vi "SendRawCommand.vi"(8 "Error In":errorcluster, 10 "Command":string, 11 "VISA resource name":refnum<visa-resource-name>) -> (0 "Error Out":errorcluster, 3 "VISA resource name out":refnum<visa-resource-name>)   [LabVIEW 2019, in "Mark 10 TSTM-DC.lvlib"]
uses:
  Mark 10 TSTM-DC.lvlib
  Mark 10 Event Monitor/Mark 10 Event Monitor.lvlib
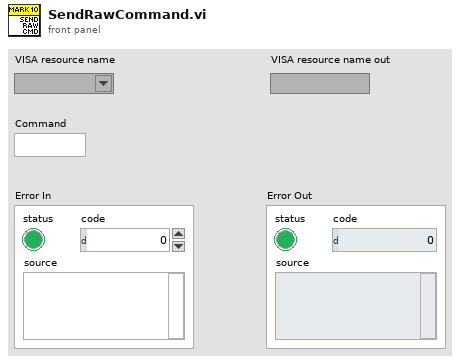
[diagram p1: front panel]
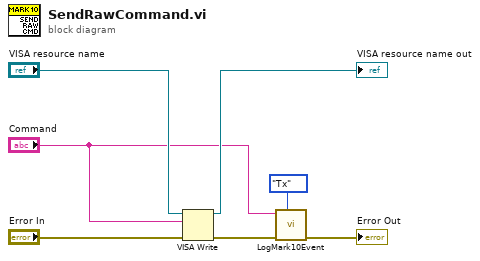
[diagram p0: block diagram]
diagram:
  n1 = VISA Write(VISA resource name="VISA resource name", write buffer="Command", error in (no error)="Error In") -> (VISA resource name out=→"VISA resource name out":refnum<visa-resource-name>, error out=w6:errorcluster)  [unwired: 1 out]
  n2 = call "LogMark10Event.vi"("Type"=enum16{"Tx", "Rx"}."Tx", "Error In"=w6, "Event"="Command") -> ("Error Out"=→"Error Out":errorcluster)  [unwired: 8 in]
